vi "校准日志.vi"(8 "error in (no error)":errorcluster, 11 "日志信息":string) -> (0 "error out":errorcluster)   [LabVIEW 2016, in "斯坦道多参数.lvlib"]
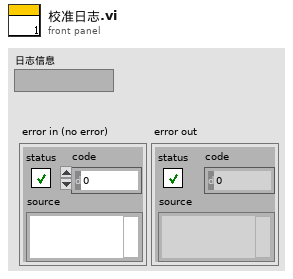
[diagram p1: front panel]
types:
  T1 = typedef "校准日志字段定义.ctl" = cluster{"时间":timestamp, "参数":string, "日志信息":string, "流程参数":string}
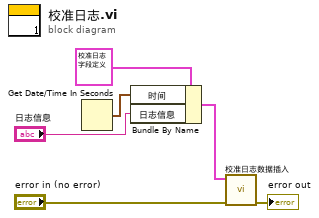
[diagram p0: block diagram]
diagram:
  n1 = Get Date/Time In Seconds() -> (seconds since 1Jan1904=w2:timestamp)
  n2 = Bundle By Name(cluster=T1 {"时间"=timestamp(0 s since 1904-01-01), "参数"="多参数", "日志信息"="", "流程参数"=""} ("data"), "时间"=w2, "日志信息"="日志信息") -> (w3:T1)
  n3 = call "校准日志数据插入.vi"("data"=w3, "错误输入（无错误）"="error in (no error)") -> ("错误输出"=→"error out":errorcluster)  [unwired: 8 in]
